vi "Add Error Core.vi"(8 "error in (no error)":errorcluster, 10 "String to Append":string, 11 "Error":T1) -> (0 "error out":errorcluster)   [LabVIEW 2021, in "ChannelCommon.lvlib"]
uses:
  ChannelCommon.lvlib
  <vilib>/CIF Foundation/CIF Utilities/Errors/Errors_CIF_U.lvlib
  typedef/Errors.ctl
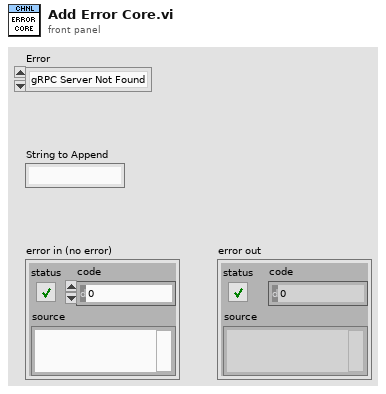
[diagram p1: front panel]
types:
  T1 = typedef "ChannelCommon.lvlib/Errors.ctl" = enum16{"gRPC Server Not Found", "Duplicate Channel", "Missing Channel", "Incorrect Type", "Flatten Error", "Unflatten Data", "Channel Length", "Plugin Connection", "gRPC Server Connection", "FIFO Unflatten", "Required Override", "Remove Not Found", "Multi Sub Not Supported", "Primary Already Connected", "Backpressure Not Supported", "Unable to Increase Buffer", "Data too Large"}
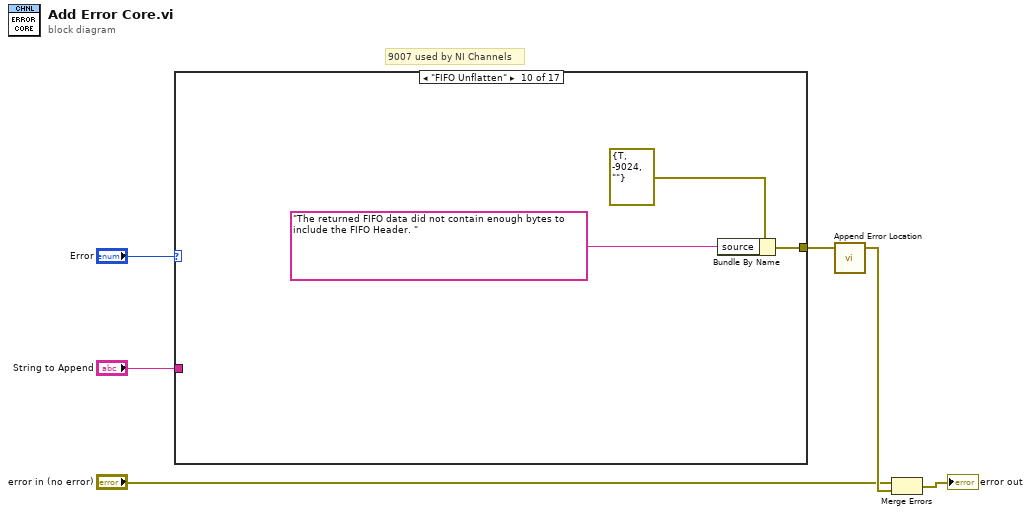
[diagram p0: block diagram]
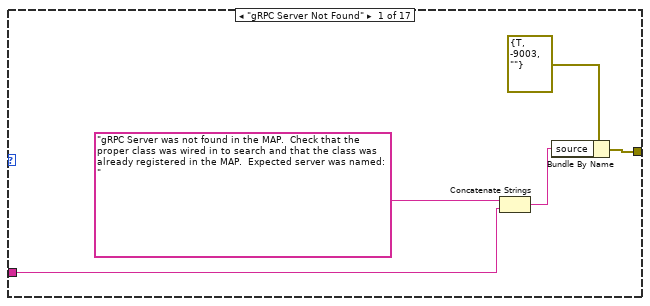
[diagram p2: hidden frame]
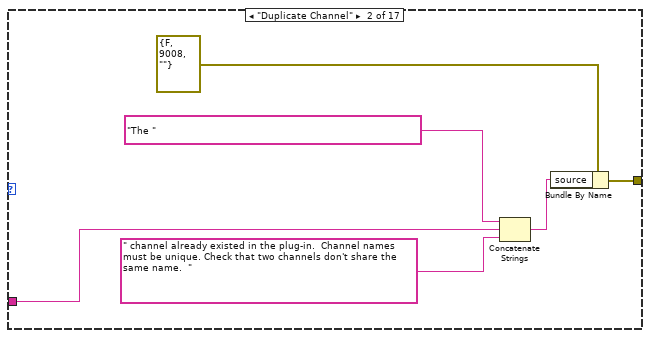
[diagram p3: hidden frame]
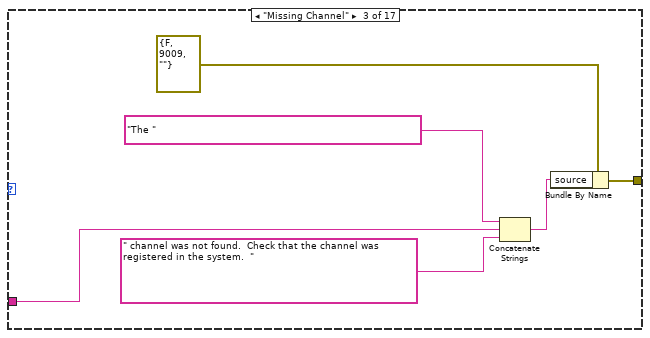
[diagram p4: hidden frame]
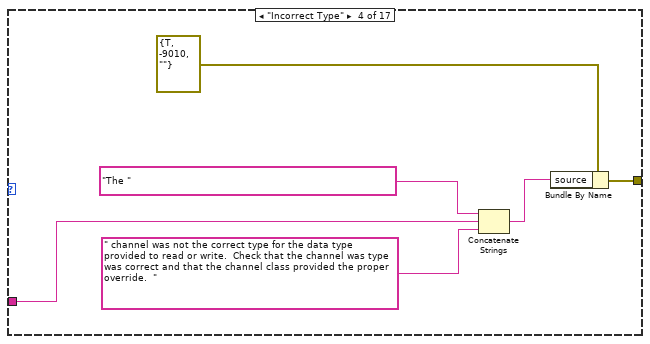
[diagram p5: hidden frame]
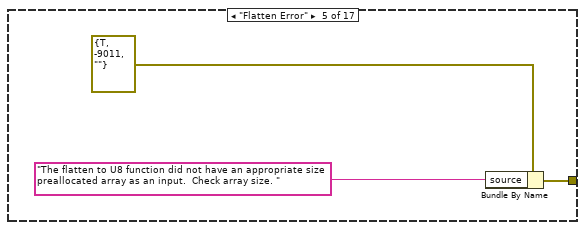
[diagram p6: hidden frame]
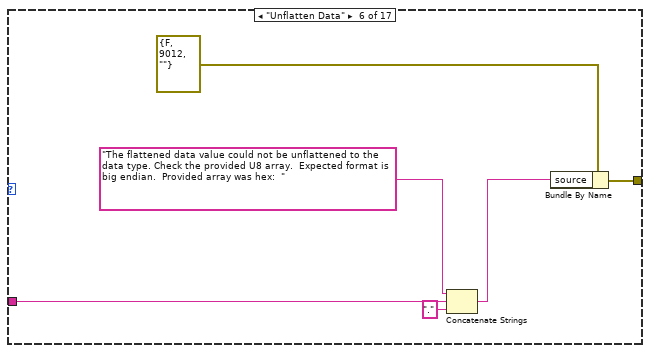
[diagram p7: hidden frame]
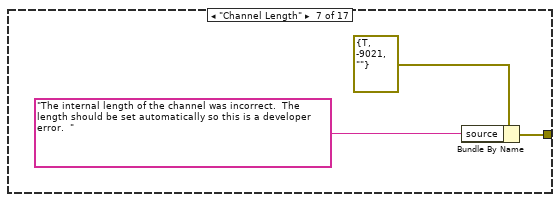
[diagram p8: hidden frame]
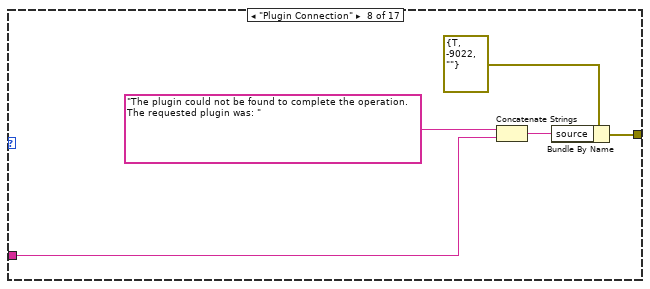
[diagram p9: hidden frame]
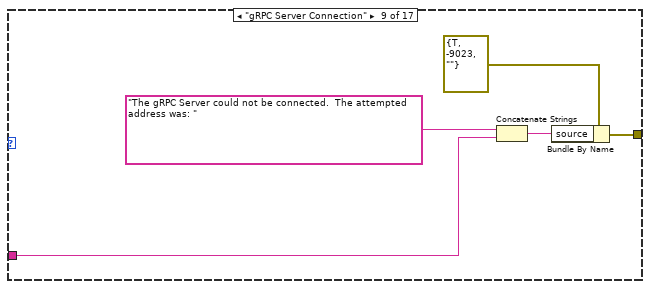
[diagram p10: hidden frame]
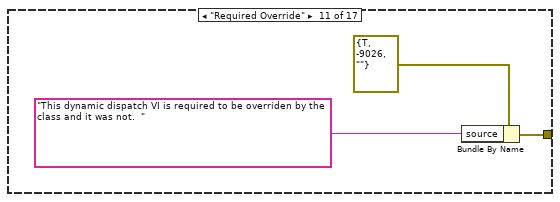
[diagram p11: hidden frame]
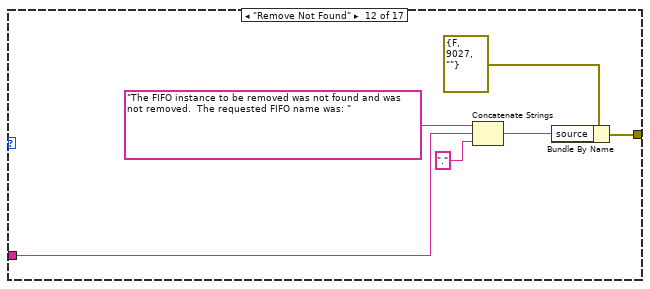
[diagram p12: hidden frame]
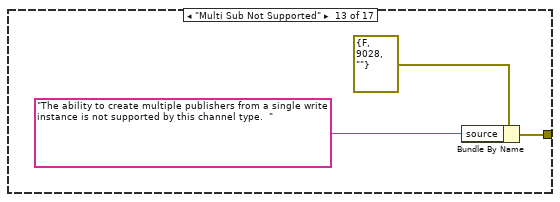
[diagram p13: hidden frame]
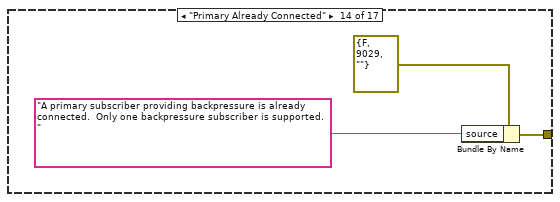
[diagram p14: hidden frame]
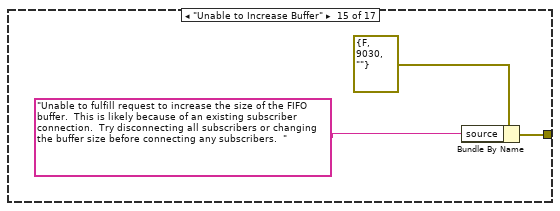
[diagram p15: hidden frame]
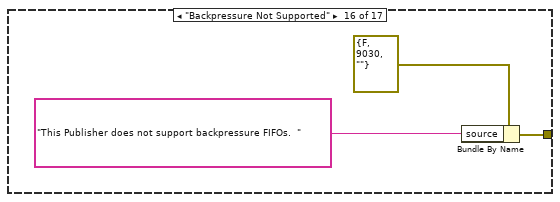
[diagram p16: hidden frame]
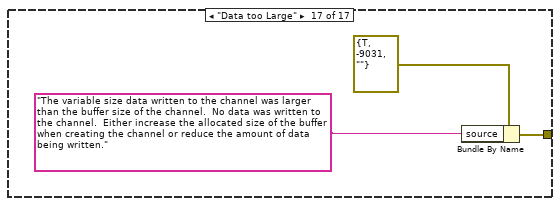
[diagram p17: hidden frame]
diagram:
  # "9007 used by NI Channels"
  n1 = case shown="\"FIFO Unflatten\"" "Error" {
    tunnel: "String to Append" -> [w8 w14 w18 w24 _ w35 _ w42 w47 _ _ w60 _ _ _ _ _]
    tunnel: [w10 w16 w22 w28 w31 w37 w40 w45 w50 w53 w56 w62 w65 w68 w71 w74 w77] -> w5
    frame "gRPC Server Not Found" {
      n2 = Concatenate Strings("gRPC Server was not found in the MAP.  Check that the proper class was wired in to search and that the class was already registered in the MAP.  Expected server was named:  " ("source"), w8) -> (w9:string)
      n3 = Bundle By Name(cluster=errorcluster {"status"=TRUE, "code"=-9003, "source"=""} ("Invalid ID"), "source"=w9) -> (w10:errorcluster)
    }
    frame "Duplicate Channel" {
      n4 = Concatenate Strings("The " ("source"), w14, " channel already existed in the plug-in.  Channel names must be unique. Check that two channels don't share the same name.  " ("source")) -> (w15:string)
      n5 = Bundle By Name(cluster=errorcluster {"status"=FALSE, "code"=9008, "source"=""} ("Invalid ID"), "source"=w15) -> (w16:errorcluster)
    }
    frame "Missing Channel" {
      n6 = Concatenate Strings("The " ("source"), w18, " channel was not found.  Check that the channel was registered in the system.  " ("source")) -> (w21:string)
      n7 = Bundle By Name(cluster=errorcluster {"status"=FALSE, "code"=9009, "source"=""} ("Invalid ID"), "source"=w21) -> (w22:errorcluster)
    }
    frame "Incorrect Type" {
      n8 = Concatenate Strings("The " ("source"), w24, " channel was not the correct type for the data type provided to read or write.  Check that the channel was type was correct and that the channel class provided the proper override.  " ("source")) -> (w25:string)
      n9 = Bundle By Name(cluster=errorcluster {"status"=TRUE, "code"=-9010, "source"=""} ("Invalid ID"), "source"=w25) -> (w28:errorcluster)
    }
    frame "Flatten Error" {
      n10 = Bundle By Name(cluster=errorcluster {"status"=TRUE, "code"=-9011, "source"=""} ("Invalid ID"), "source"="The flatten to U8 function did not have an appropriate size preallocated array as an input.  Check array size. ") -> (w31:errorcluster)
    }
    frame "Unflatten Data" {
      n11 = Concatenate Strings("The flattened data value could not be unflattened to the data type. Check the provided U8 array.  Expected format is big endian.  Provided array was hex:  " ("source"), w35, "." ("string")) -> (w33:string)
      n12 = Bundle By Name(cluster=errorcluster {"status"=FALSE, "code"=9012, "source"=""} ("Invalid ID"), "source"=w33) -> (w37:errorcluster)
    }
    frame "Channel Length" {
      n13 = Bundle By Name(cluster=errorcluster {"status"=TRUE, "code"=-9021, "source"=""} ("Invalid ID"), "source"="The internal length of the channel was incorrect.  The length should be set automatically so this is a developer error.  ") -> (w40:errorcluster)
    }
    frame "Plugin Connection" {
      n14 = Concatenate Strings("The plugin could not be found to complete the operation.  The requested plugin was: " ("source"), w42) -> (w43:string)
      n15 = Bundle By Name(cluster=errorcluster {"status"=TRUE, "code"=-9022, "source"=""} ("Invalid ID"), "source"=w43) -> (w45:errorcluster)
    }
    frame "gRPC Server Connection" {
      n16 = Concatenate Strings("The gRPC Server could not be connected.  The attempted address was: " ("source"), w47) -> (w48:string)
      n17 = Bundle By Name(cluster=errorcluster {"status"=TRUE, "code"=-9023, "source"=""} ("Invalid ID"), "source"=w48) -> (w50:errorcluster)
    }
    frame "FIFO Unflatten" {
      n18 = Bundle By Name(cluster=errorcluster {"status"=TRUE, "code"=-9024, "source"=""} ("Invalid ID"), "source"="The returned FIFO data did not contain enough bytes to include the FIFO Header. ") -> (w53:errorcluster)
    }
    frame "Required Override" {
      n19 = Bundle By Name(cluster=errorcluster {"status"=TRUE, "code"=-9026, "source"=""} ("Invalid ID"), "source"="This dynamic dispatch VI is required to be overriden by the class and it was not.  ") -> (w56:errorcluster)
    }
    frame "Remove Not Found" {
      n20 = Concatenate Strings("The FIFO instance to be removed was not found and was not removed.  The requested FIFO name was: " ("source"), w60, "." ("string")) -> (w58:string)
      n21 = Bundle By Name(cluster=errorcluster {"status"=FALSE, "code"=9027, "source"=""} ("Invalid ID"), "source"=w58) -> (w62:errorcluster)
    }
    frame "Multi Sub Not Supported" {
      n22 = Bundle By Name(cluster=errorcluster {"status"=FALSE, "code"=9028, "source"=""} ("Invalid ID"), "source"="The ability to create multiple publishers from a single write instance is not supported by this channel type.  ") -> (w65:errorcluster)
    }
    frame "Primary Already Connected" {
      n23 = Bundle By Name(cluster=errorcluster {"status"=FALSE, "code"=9029, "source"=""} ("Invalid ID"), "source"="A primary subscriber providing backpressure is already connected.  Only one backpressure subscriber is supported.  ") -> (w68:errorcluster)
    }
    frame "Unable to Increase Buffer" {
      n24 = Bundle By Name(cluster=errorcluster {"status"=FALSE, "code"=9030, "source"=""} ("Invalid ID"), "source"="Unable to fulfill request to increase the size of the FIFO buffer.  This is likely because of an existing subscriber connection.  Try disconnecting all subscribers or changing the buffer size before connecting any subscribers.  ") -> (w71:errorcluster)
    }
    frame "Backpressure Not Supported" {
      n25 = Bundle By Name(cluster=errorcluster {"status"=FALSE, "code"=9030, "source"=""} ("Invalid ID"), "source"="This Publisher does not support backpressure FIFOs.  ") -> (w74:errorcluster)
    }
    frame "Data too Large" {
      n26 = Bundle By Name(cluster=errorcluster {"status"=TRUE, "code"=-9031, "source"=""} ("Invalid ID"), "source"="The variable size data written to the channel was larger than the buffer size of the channel.  No data was written to the channel.  Either increase the allocated size of the buffer when creating the channel or reduce the amount of data being written.") -> (w77:errorcluster)
    }
  }
  n27 = call <vilib>:"Append Error Location.vi"("error in (no error)"=w5) -> ("error out"=w6:errorcluster)  [unwired: 4 in]
  n28 = Merge Errors("error in (no error)", w6) -> (→"error out":errorcluster)
